vi "Build XML tag.vi"(10 "Alias":string) -> (2 "XML Tag":string)   [LabVIEW 2020]
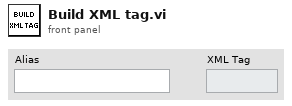
[diagram p1: front panel]
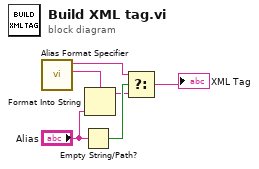
[diagram p0: block diagram]
diagram:
  n1 = call "Alias Format Specifier.vi"() -> ("Alias Format specifier"=w4:string, "Default Alias"=w3:string)  [unwired: 10 in]
  n2 = Empty String/Path?(string/path="Alias") -> (empty?=w6:bool)
  n3 = Format Into String(format string=w4, "Alias") -> (resulting string=w5:string)  [unwired: 2 in, 1 out]
  n4 = Select(t=w3, s=w6, f=w5) -> (s? t:f=→"XML Tag":string)
